vi "From Double.vi"(8 "error in (no error)":errorcluster, 10 "Double":dbl) -> (0 "error out":errorcluster, 3 "Double Scalar SensorData out":refnum<class "Double Scalar SensorData.lvclass">)   [LabVIEW 2012, in "Sensor Definition.lvlib" / "Double Scalar SensorData.lvclass"]
uses:
  Double Scalar SensorData.lvclass
  Double Scalar SensorData.lvclass/Double Scalar SensorData.ctl
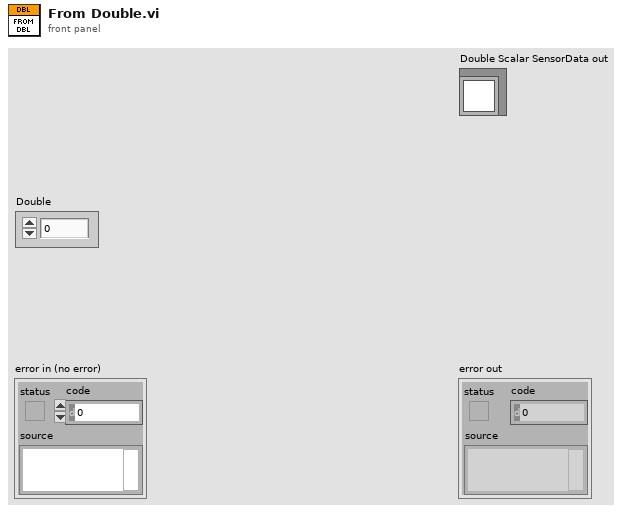
[diagram p1: front panel]
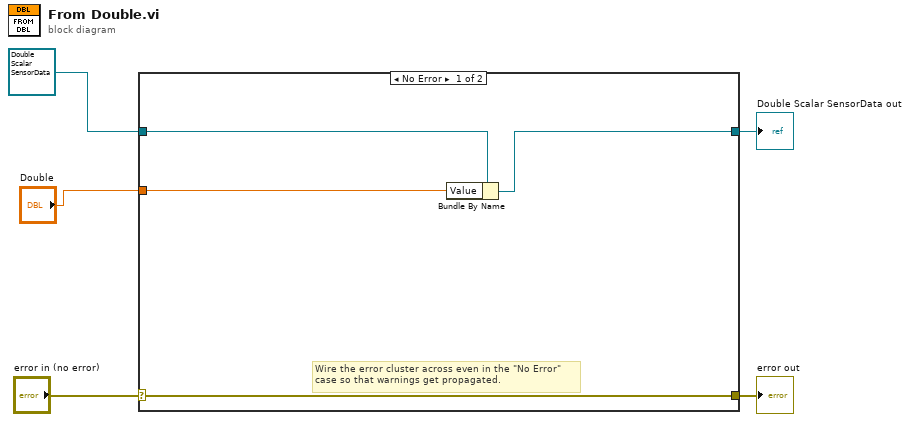
[diagram p0: block diagram]
diagram:
  n1 = case shown="No Error" "error in (no error)" {
    selector: "error in (no error)" -> [w9 w11]
    tunnel: [w9 w11] -> w4
    tunnel: [w7 w10] -> w2
    tunnel: refnum<class "Double Scalar SensorData.lvclass"> refnum ("Double Scalar SensorData in") -> [w8 w10]
    tunnel: "Double" -> [w6 _]
    frame No Error {
      # "Wire the error cluster across even in the \"No Error\"\ncase so that warnings get propagated."
      n2 = Bundle By Name(cluster=w8, "Value"=w6) -> (w7:refnum<class "Double Scalar SensorData.lvclass">)
    }
    frame Error {
    }
  }
  "error out" <- w4
  "Double Scalar SensorData out" <- w2
